vi "generateRampedSquareWave.vi"(0 "pulses":dbl, 1 "phase shift(ms)":dbl, 4 "Period (ms)":dbl, 5 "Repeats":dbl, 6 "Sampling frequency (Hz)":dbl, 7 "Cycles":dbl, 8 "DC (%)":dbl, 9 "Step size (V)":dbl, 10 "Baseline (V)":dbl, 11 "Start amplitude (V)":dbl) -> (2 "wflength":i32, 3 "Waveform":waveform(dbl))   [LabVIEW 2015]
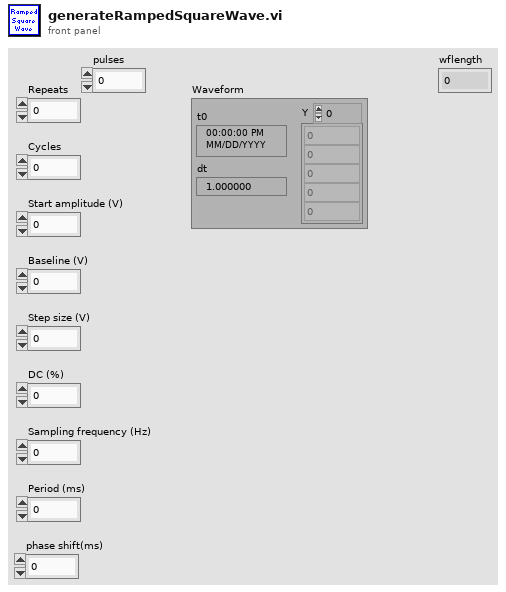
[diagram p1: front panel]
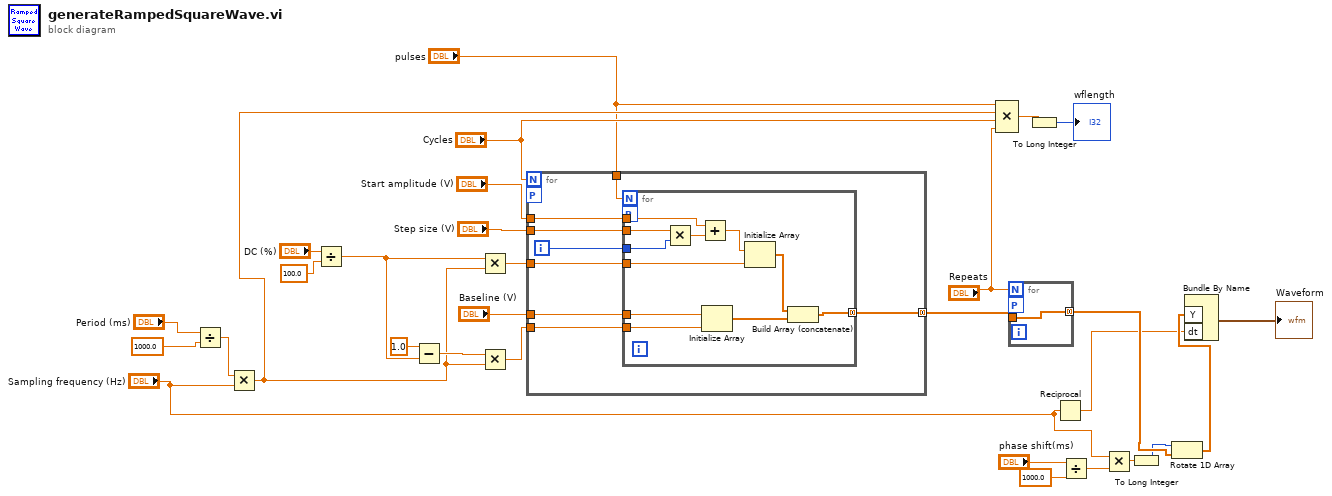
[diagram p0: block diagram]
diagram:
  n1 = Divide(x="Period (ms)", y=1000.0) -> (x/y=w16:dbl)
  n2 = Multiply(x=w16, y="Sampling frequency (Hz)") -> (x*y=w13:dbl)
  n3 = Divide(x="DC (%)", y=100.0) -> (x/y=w25:dbl)
  n4 = Subtract(x=1.0, y=w25) -> (x-y=w23:dbl)
  n5 = Multiply(x=w25, y=w13) -> (x*y=w26:dbl)
  n6 = Multiply(x=w23, y=w13) -> (x*y=w24:dbl)
  n7 = for {
    N: "Cycles" -> [_]
    tunnel: w24 -> [w38]
    tunnel: w26 -> [w37]
    tunnel: "Start amplitude (V)" -> [w34]
    tunnel: "Step size (V)" -> [w33]
    tunnel: "Baseline (V)" -> [w32]
    tunnel: [w35] -> w17 mode=concatenating
    workers-P: _ -> [_]
    tunnel: "pulses" -> [w31]
    i -> [w36]
    n8 = for {
      N: w31 -> [_]
      tunnel: w38 -> [w49]
      tunnel: w37 -> [w48]
      tunnel: w36 -> [w46]
      tunnel: [w44] -> w35 mode=concatenating
      tunnel: w34 -> [w41]
      tunnel: w33 -> [w40]
      tunnel: w32 -> [w39]
      workers-P: _ -> [_]
      n9 = Multiply(x=w40, y=w46) -> (x*y=w47:dbl)
      n10 = Add(x=w41, y=w47) -> (x+y=w45:dbl)
      n11 = Initialize Array(w39, w49) -> (w42:dbl[])
      n12 = Initialize Array(w45, w48) -> (w43:dbl[])
      n13 = Build Array (concatenate)(w43, w42) -> (w44:dbl[])
    }
  }
  n14 = Compound Arithmetic op=MULTIPLY("pulses", w13, "Cycles", "Repeats") -> (w12:dbl)
  n15 = for {
    N: "Repeats" -> [_]
    workers-P: _ -> [_]
    tunnel: w17 -> [w50]
    tunnel: [w50] -> w7 mode=concatenating
  }
  n16 = To Long Integer(number=w12) -> (32bit integer=→"wflength":i32)
  n17 = Reciprocal(x="Sampling frequency (Hz)") -> (1/x=w2:dbl)
  n18 = Divide(x="phase shift(ms)", y=1000.0) -> (x/y=w8:dbl)
  n19 = Multiply(x="Sampling frequency (Hz)", y=w8) -> (x*y=w6:dbl)
  n20 = To Long Integer(number=w6) -> (32bit integer=w5:i32)
  n21 = Rotate 1D Array(1:w7, 2:w5) -> (0:w4:dbl[])
  n22 = Bundle By Name("Y"=w4, "dt"=w2) -> (→"Waveform":waveform(dbl))  [unwired: 1 in]
